vi "RF_Attn_move.vi"(1 "Points":cluster{string, "data":u64, "data":dbl}, 2 "Instr. Info":T1) -> ()   [LabVIEW 2013]
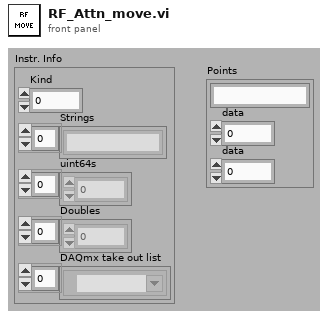
[diagram p1: front panel]
types:
  T1 = cluster{"Kind":u16, "Strings":string[], "uint64s":u64[], "Doubles":dbl[], "DAQmx take out list":refnum<k21>[]}
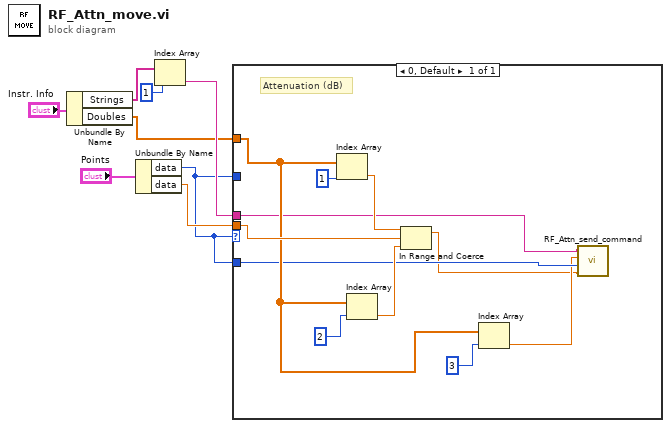
[diagram p0: block diagram]
diagram:
  n1 = Unbundle By Name("Instr. Info") -> ("Strings"=w6:string[], "Doubles"=w2:dbl[])
  n2 = Unbundle By Name("Points") -> ("data"=w1:u64, "data"=w3:dbl)
  n3 = Index Array(array=w6, index=1) -> (element=w4:string)
  n4 = case shown="0, Default" w1 {
    tunnel: w4 -> [w12]
    tunnel: w3 -> [w17]
    tunnel: w1 -> [_]
    tunnel: w2 -> [w13]
    tunnel: w1 -> [w11]
    frame 0, Default {
      # "Attenuation (dB)"
      n5 = Index Array(array=w13, index=1) -> (element=w16:dbl)
      n6 = Index Array(array=w13, index=2) -> (element=w15:dbl)
      n7 = In Range and Coerce(upper limit=w16, x=w17, lower limit=w15) -> (coerced(x)=w9:dbl)  [unwired: 1 out]
      n8 = Index Array(array=w13, index=3) -> (element=w10:dbl)
      n9 = call "RF_Attn_send_command.vi"("Value"=w9, "Parameter"=w11, "Insertion Loss"=w10, "USB address"=w12) -> ()  [unwired: 1 in]
    }
  }
